vi "SetMotorParameters.vi"(0 "handle in":i32, 1 "UnitAddress(0)":u16, 2 "MotNr(0)":u8, 5 "error in":errorcluster, 7 "Motor Parameter":T1={"Poslimit (6400)"=6400, "P5 Bits"={"MT_PI"=FALSE, "MT_ROTARY"=FALSE, "MT_AUTONULLCMD"=FALSE, "MT_TESTNULL"=FALSE, "MT_NULLLEFT"=FALSE, "MT_NULLCENTRE"=TRUE, "MT_STOPNULL"=FALSE, "MT_FILTERSWITCH"=TRUE}, "P6 Bits"={"MT_OPTIMIZEWAY"=FALSE, "MT_FASTREF"=TRUE, "MT_MECHREF"=FALSE, "MT_DELAYTESTNULL"=TRUE, "MT_STOPSOFT"=FALSE, "MT_STOPNOREF"=FALSE, "MT_NULLPOSITIVE"=FALSE, "MUT_STOPFULSTEPS"=FALSE}} {"Poslimit (6400)" step=1}) -> (14 "handle out":i32, 19 "error out":errorcluster)   [LabVIEW 2014, in "Sixpack - Driver.lvlib"]
doc: "CMD $15\nMotorNr (0...5)\nPoslimit: Bei rotatorischen Achsen: Mikroschritte pro Umdrehung (Vollschritte * 16). Bei linearen Achsen (MT_ROTARY = 0): Mindestens der gesamte Fahrbereich, um ungewollte oder unterbrochene Referenzfahrten zu vermeiden!\n\nMotorType (untere acht Bits):\nBit0: MT_PI\n0 = Rampenfahrt (Default)\n1 = PI-Regler\nBit1: MT_ROTARY\n0 = lineare Achse (Default)\n1 = rotatorische Achse\nBit2: MT_AUTONULLCMD\n1 = nach Senden des Befehls wird Referenzfahrt durchgeführt (siehe auch ReferenceSearch)\nBit3: MT_TESTNULL\n1 = Wenn interner Positionszähler auf Position des Referenzpunktes, Referenzschalter jedoch nicht aktiv wird STOPFLAG (siehe GetPositionAndActivity) gesetzt. Es folgt eine Referenzfahrt wenn MT_STOPNOREF nicht gesetzt. Wird nur bei stehendem Motor überprüft!\nBit4: MT_NULLLEFT\n0 = Referenzpunkt rechts vom Fahrbereich\n1 = Referenzpunkt links vom Fahrbereich\nBit5: MT_NULLCENTRE\n1 = Referenzpunkt wird in der Mitte des Aktivitätsbereiches des Referenzschalters gesucht. Ist für rotatorische Achsen besonders sinnvoll. (Default)\nBit6: MT_STOPNULL\n1 = Definiert den Referenzschalter als Endschalter (Achsenseite wird durch MT_NULLEFT definiert). Wenn Referenzschalter aktiviert, wird STOPFLAG gesetzt (siehe GetPositionAndActivity). Zudem wird überprüft, ob Status des Referenzschalters und Wert des internen Positionszählers gemeinsam gültig sind. Wenn nicht und MT_STOPNOREF=0 wird eine Referenzfahrt durchgeführt\nBit7: MT_FILTERSWITCH\n1 = Referenzschalter wird per Software entprellt (siehe SetRefSearchParameters, Variable DebouncingTime) (Default) \n\nMotorType (obere acht Bits):\nBit0: MT_OPTIMIZEWAY\n1 = Wegoptimierung für rotatorische Achsen durch Auswahl von Links-/Rechtslauf \nBit1: MT_FASTREF\n1 = Referenzfahrt mit hoher Geschwindigkeit (siehe SetRefSearchParameters) (default)\nBit2: MT_MECHREF\n1 = Mechanischer Anschlag für Referenzfahrt (siehe Kapitel 2.5.1)\nBit3: MT_DELAYTESTNULL\n1 = Zustand des Referenzschalters und interner Positionszähler werden um die in der Variablen PowerDownDelay (siehe SetCurrentControl) gesetzte Zeit verzögert verglichen. Dies verhindert Fehler durch Ungenauigkeiten in der Mechanik in Verbindung mit MT_TESTNULL. (default)\nBit4: MT_STOPSOFT\n0 = Motor wird bei Eintreten von Stopp- Bedingung (Endschalter aktiviert) abrupt gestoppt. Da es hierbei zu Schrittverlusten kommen kann, schließt sich eine Referenzfahrt an. Die kann durch setzen von MT_STOPNOREF verhindert werden. \n1= Motor wird bei Eintreten von Stopp- Bedingung mit einer negativen Beschleunigung vom Betrag AMax abgebremst. Sollte die Stopp-Bedingung vor dem Stillstand aufgehoben werden, wird der vorangegangene Fahrbefehl weiter ausgeführt.\nBit5: MT_STOPNOREF\n1 = Es wird keine automatische Referenzfahrt ausgeführt, wenn Stopp-Bedingung eingetreten.\nBit6: MT_NULLPOSITIVE\n0 = Referenzeingang ist low aktiv (Schalter ist Schließer)\n1 = Referenzschalter ist high aktiv (Schalter ist Öffner)\nBit7: MT_STOPFULLSTEPS\n1 = Fahrrampen werden so berechnet, dass sie nur an Vollschrittpositionen enden \n\nACHTUNG: Einige Flags sind in der Standarteinstellung schon gesetzt (siehe „Default“ in der Beschreibung hier oder Kapitel 3.7). D.h. diese Funktionen sind von Beginn an aktiviert. Wird nun SetMotorParameters aufgerufen, werden alle Flags so wie in der Variablen MotorType angegeben, gesetzt.\n\nPACK_DLL: Der Parameter MotorType sollte aus den Konstanten MT_xxx aus dem Headerfile durch verodern gebildet werden."
uses:
  Sixpack - Driver.lvlib
  Motor Parameter.ctl
  MotorParameter_P5.ctl
  MotorParameter_P6.ctl
  DLL/PackDLL.dll
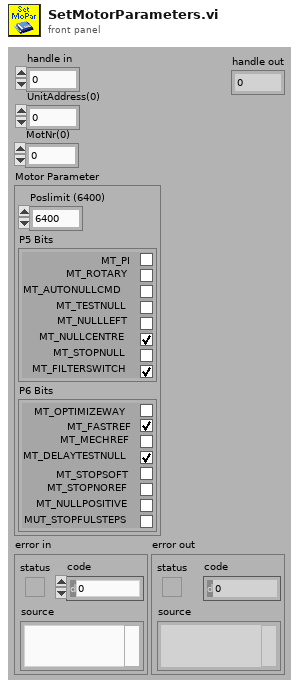
[diagram p1: front panel]
types:
  T1 = typedef "Sixpack - Driver.lvlib/Motor Parameter.ctl" = cluster{"Poslimit (6400)":u32, "P5 Bits":T2, "P6 Bits":T3}
  T2 = typedef "Sixpack - Driver.lvlib/MotorParameter_P5.ctl" = cluster{"MT_PI":bool, "MT_ROTARY":bool, "MT_AUTONULLCMD":bool, "MT_TESTNULL":bool, "MT_NULLLEFT":bool, "MT_NULLCENTRE":bool, "MT_STOPNULL":bool, "MT_FILTERSWITCH":bool}
  T3 = typedef "Sixpack - Driver.lvlib/MotorParameter_P6.ctl" = cluster{"MT_OPTIMIZEWAY":bool, "MT_FASTREF":bool, "MT_MECHREF":bool, "MT_DELAYTESTNULL":bool, "MT_STOPSOFT":bool, "MT_STOPNOREF":bool, "MT_NULLPOSITIVE":bool, "MUT_STOPFULSTEPS":bool}
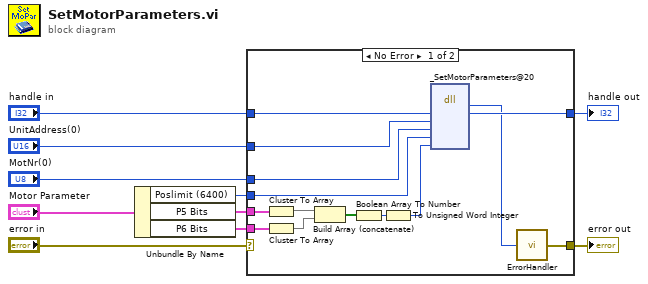
[diagram p0: block diagram]
diagram:
  n1 = Unbundle By Name("Motor Parameter") -> ("Poslimit (6400)"=w3:u32, "P5 Bits"=w2:T2, "P6 Bits"=w1:T3)
  n2 = case shown="No Error" "error in" {
    selector: "error in" -> [_ w25]
    tunnel: "handle in" -> [w24 w26]
    tunnel: [w23 w26] -> w9
    tunnel: "UnitAddress(0)" -> [w22 _]
    tunnel: "MotNr(0)" -> [w21 _]
    tunnel: w3 -> [w20 _]
    tunnel: [w13 w25] -> w5
    tunnel: w2 -> [w12 _]
    tunnel: w1 -> [w11 _]
    frame No Error {
      n3 = Cluster To Array(cluster=w12) -> (array=w19:bool[])
      n4 = Cluster To Array(cluster=w11) -> (array=w18:bool[])
      n5 = Build Array (concatenate)(w19, w18) -> (w17:bool[])
      n6 = Boolean Array To Number(Boolean array=w17) -> (number=w16:u32)
      n7 = To Unsigned Word Integer(number=w16) -> (unsigned 16bit integer=w15:u16)
      n8 = dll-call lib="D:/CS-Source/LV2014/GPL/instr.lib/SixPack/PackDLL/DLL/PackDLL.dll" fn="_SetMotorParameters@20" label="SetMotorParameters"("HANDLE"=w24, "UnitAddress"=w22, "MotNr"=w21, "PosLimit"=w20, "MotorType"=w15) -> ("BOOLEAN"=w14:i8, "HANDLE"=w23:i32)  [unwired: 7 in, 2 out]
      n9 = call "ErrorHandler.vi"("BOOLEAN"=w14) -> ("error out"=w13:errorcluster)
    }
    frame Error {
    }
  }
  "handle out" <- w9
  "error out" <- w5
